vi "例程02-加减乘除.vi"() -> ()   [LabVIEW 2021]
panel:
  out "结果*":dbl
  out "结果/":dbl
  out "结果-":dbl
  out "结果+":dbl
  in  "输入2":dbl
  in  "输入1":dbl
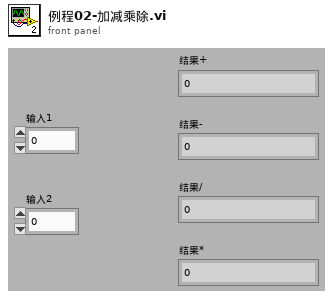
[diagram p1: front panel]
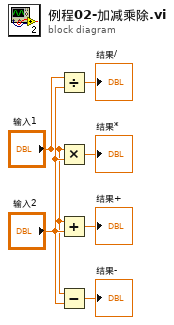
[diagram p0: block diagram]
diagram:
  n1 = Divide(x="输入1", y="输入2") -> (x/y=→"结果/":dbl)
  n2 = Multiply(x="输入1", y="输入2") -> (x*y=→"结果*":dbl)
  n3 = Add(x="输入1", y="输入2") -> (x+y=→"结果+":dbl)
  n4 = Subtract(x="输入1", y="输入2") -> (x-y=→"结果-":dbl)
